vi "SetGetSystemSettings - Test.vi"() -> ()   [LabVIEW 2017]
uses:
  AT901 API/Structures/Struct SystemSettingsData.ctl
  AT901 API/TypeDefinitions/ES_WeatherMonitorStatus.ctl
panel:
  in  "SystemSettingsData":T1={"WeatherMonitorStatus"=enum."ES_WMS_ReadAndCalculateRefractions", "ApplyTransformationParams"=FALSE, "ApplyStationOrientationParams"=FALSE, "KeepLastPosition"=TRUE, "SendUnsolicitedMessages"=TRUE, "SendReflectorPositionData"=FALSE, "TryMeasurementMode"=FALSE, "HasNivel"=FALSE, "HasVideoCamera"=FALSE}
  out "SystemSettingsData OUT":T1
  out "error out":errorcluster
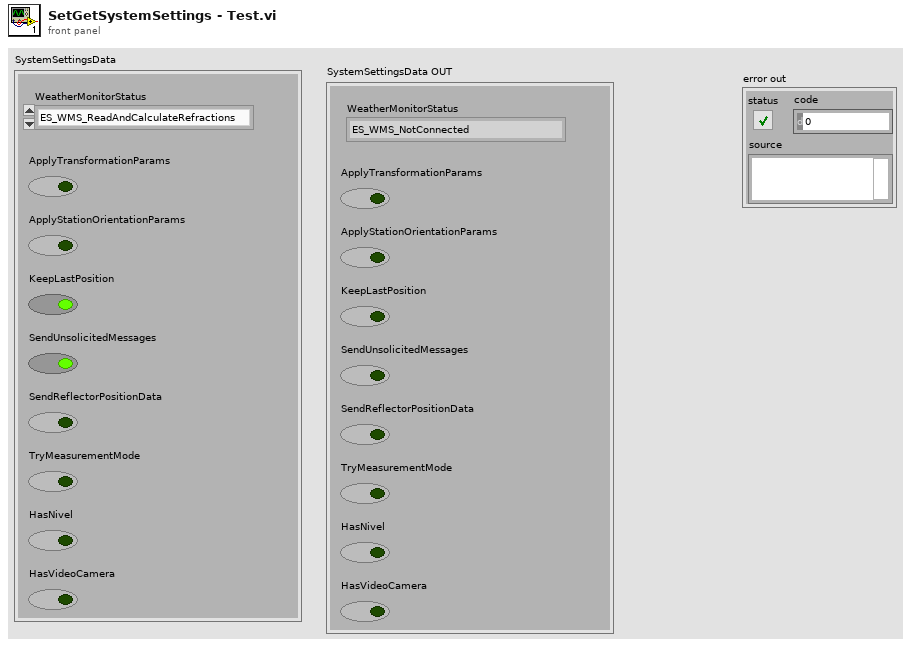
[diagram p1: front panel]
types:
  T1 = typedef "Struct SystemSettingsData.ctl" = cluster{"WeatherMonitorStatus":T2, "ApplyTransformationParams":bool, "ApplyStationOrientationParams":bool, "KeepLastPosition":bool, "SendUnsolicitedMessages":bool, "SendReflectorPositionData":bool, "TryMeasurementMode":bool, "HasNivel":bool, "HasVideoCamera":bool}
  T2 = typedef "ES_WeatherMonitorStatus.ctl" = enum16{"ES_WMS_NotConnected", "ES_WMS_ReadOnly", "ES_WMS_ReadAndCalculateRefractions"}
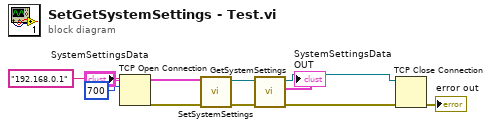
[diagram p0: block diagram]
diagram:
  n1 = TCP Open Connection(address="192.168.0.1", remote port or service name=u16 700) -> (connection ID=w4:refnum<k5>, error out=w1:errorcluster)  [unwired: 3 in]
  n2 = call "SetSystemSettings.vi"("error in (no error)"=w1, "SystemSettingsData"="SystemSettingsData", "TCP Network Connection in"=w4) -> ("error out"=w2:errorcluster, "TCP Network Connection out"=w3:refnum<k5>)  [unwired: 5 in, 2 out]
  n3 = call "GetSystemSettings.vi"("error in (no error)"=w2, "TCP Network Connection in"=w3) -> ("error out"=w7:errorcluster, "SystemSettingsData"=→"SystemSettingsData OUT":T1, "TCP Network Connection out"=w8:refnum<k5>)  [unwired: 5 in, 2 out]
  n4 = TCP Close Connection(connection ID=w8, error in (no error)=w7) -> (error out=→"error out":errorcluster)  [unwired: 1 in, 1 out]
